vi "Configure Mechanical Attenuator List.vi"(8 "error in (no error)":errorcluster, 10 "Mechanical Attenuator List":dbl[](array[numeric])=[10.0, 10.0, 10.0], 11 "VISA resource name":refnum<visa-resource-name>) -> (0 "error out":errorcluster, 3 "VISA resource name out":refnum<visa-resource-name>)   [LabVIEW 2014, in "Agilent MXA Series.lvlib"]
doc: "Cofigures the Mechanical Attenuator List under List Sweep measurement type."
uses:
  Agilent MXA Series.lvlib
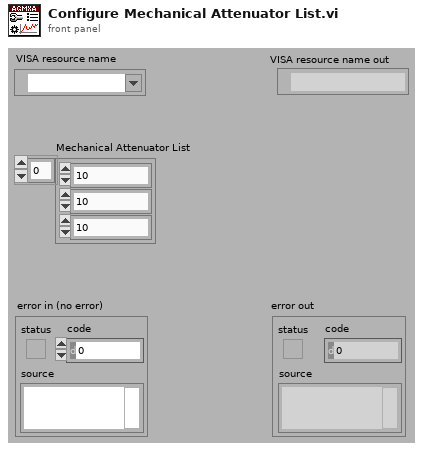
[diagram p1: front panel]
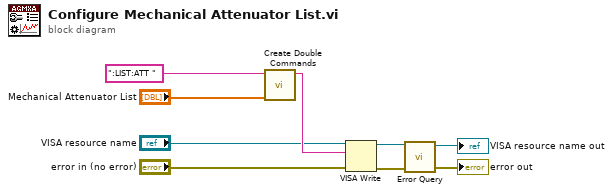
[diagram p0: block diagram]
diagram:
  n1 = call "Create Double Commands.vi"("Double Values"="Mechanical Attenuator List", "Commands"=":LIST:ATT ") -> ("Result"=w3:string)  [unwired: 9 in]
  n2 = VISA Write(VISA resource name="VISA resource name", write buffer=w3, error in (no error)="error in (no error)") -> (VISA resource name out=w6:refnum<visa-resource-name>, error out=w7:errorcluster)  [unwired: 1 out]
  n3 = call "Error Query.vi"("error in (no error)"=w7, "VISA resource name"=w6) -> ("error out"=→"error out":errorcluster, "VISA resource name out"=→"VISA resource name out":refnum<visa-resource-name>)  [unwired: 6 in, 2 out]
